vi "TDC_getDataLost.vi"(8 "Error In":errorcluster) -> (0 "Error Out":errorcluster, 3 "Data Loss":bool)   [LabVIEW 2011]
uses:
  dist/userlib/lib/tdcbase.dll
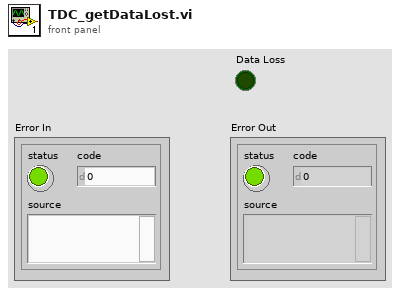
[diagram p1: front panel]
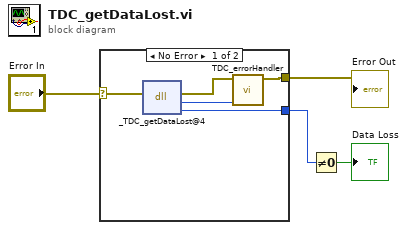
[diagram p0: block diagram]
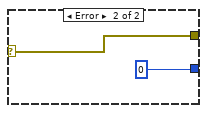
[diagram p2: hidden frame]
diagram:
  n1 = case shown="No Error" "Error In" {
    selector: "Error In" -> [w9 w11]
    tunnel: [w6 w11] -> w3
    tunnel: [w5 0] -> w1
    frame No Error {
      n2 = dll-call lib="C:/nh/projekt/spmctrl/dist/userlib/lib/tdcbase.dll" fn="_TDC_getDataLost@4"(error in=w9) -> (error out=w8:errorcluster, "return type"=w7:i32, "dataLost"=w5:i32)  [unwired: 3 in, 1 out]
      n3 = call "TDC_errorHandler.vi"("quTAU Return Code"=w7, "Error In"=w8) -> ("Error Out"=w6:errorcluster)  [unwired: 9 in]
    }
    frame Error {
    }
  }
  "Error Out" <- w3
  n4 = Not Equal To 0?(x=w1) -> (x != 0?=→"Data Loss":bool)
